vi "温度报警系统（保存到excel）.vi"() -> ()   [LabVIEW 2018]
uses:
  <vilib>/Utility/file.llb/Write Delimited Spreadsheet (string).vi
  <vilib>/Utility/file.llb/Write Delimited Spreadsheet (DBL).vi
panel:
  out "波形图表":dbl(graph)
  out "布尔":bool
  in  "预警值":dbl=50.0
  out "温度计":dbl(slide) scale=0.0..100.0
  in  "停止":bool
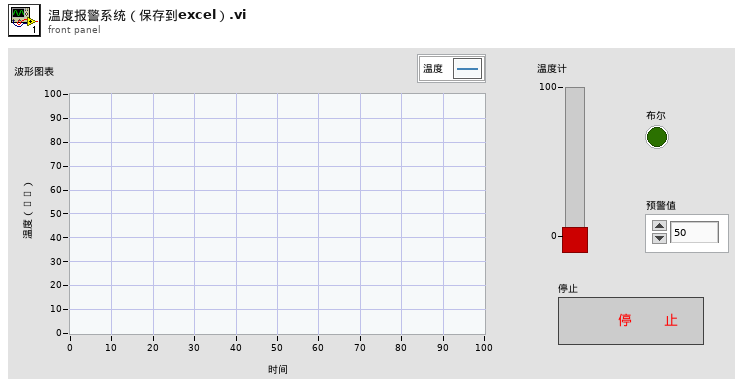
[diagram p1: front panel]
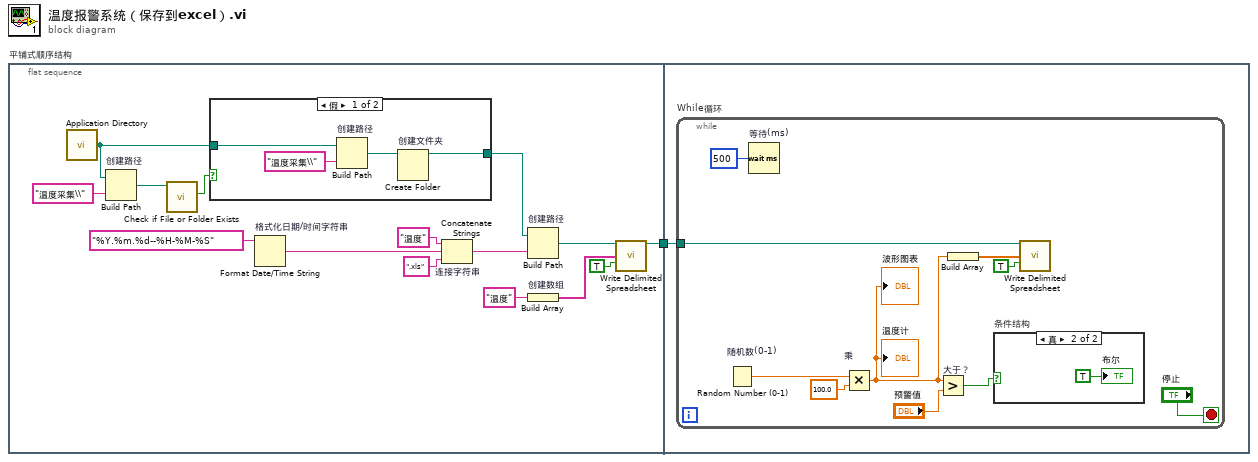
[diagram p0: block diagram]
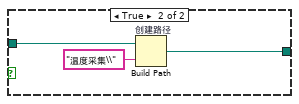
[diagram p2: hidden frame]
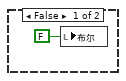
[diagram p3: hidden frame]
diagram:
  n1 = flat-sequence "平铺式顺序结构" {
    tunnel: [w3] -> w1
    tunnel: w1 -> [w24]
    frame #0 {
      n2 = call <vilib>:"Application Directory.vi"() -> ("Application Directory"=w14:path)
      n3 = Build Path "创建路径"(base path=w14, name or relative path="温度采集\\" ("名称或相对路径")) -> (appended path=w12:path)
      n4 = call <vilib>:"Check if File or Folder Exists.vi"("path"=w12) -> ("file or folder exists?"=w13:bool)  [unwired: 8 in, 2 out]
      n5 = case shown="假" w13 {
        tunnel: w14 -> [w20 w23]
        tunnel: [w17 w21] -> w7
        frame False {
          n6 = Build Path "创建路径"(base path=w20, name or relative path="温度采集\\" ("名称或相对路径")) -> (appended path=w18:path)
          n7 = Create Folder "创建文件夹"(path (use dialog)=w18) -> (created path=w17:path)  [unwired: 2 in, 2 out]
        }
        frame True {
          n8 = Build Path "创建路径"(base path=w23, name or relative path="温度采集\\" ("名称或相对路径")) -> (appended path=w21:path)
        }
      }
      n9 = Format Date/Time String "格式化日期/时间字符串"(time format string (%c)="%Y.%m.%d--%H-%M-%S" ("时间格式字符串(%c)")) -> (date/time string=w15:string)  [unwired: 2 in]
      n10 = Concatenate Strings "连接字符串"("温度" ("字符串"), w15, ".xls" ("字符串")) -> (w16:string)
      n11 = Build Path "创建路径"(base path=w7, name or relative path=w16) -> (appended path=w4:path)
      n12 = Build Array "创建数组"("温度" ("字符串")) -> (w5:string[])
      n13 = call-poly <vilib>:"Write Delimited Spreadsheet.vi"("file path (dialog if empty)"=w4, "1D data"=w5, "append to file? (new file:F)"=TRUE) -> ("new file path (Not A Path if cancelled)"=w3:path)  [unwired: 11 in, 1 out]
    }
    frame #1 {
      n14 = while "While循环" {
        tunnel: w24 -> [w28]
        stop <- "停止" stop-if-true
        n15 = Random Number (0-1) "随机数(0-1)"() -> (number: 0 to 1=w32:dbl)
        n16 = Wait (ms) "等待(ms)"(milliseconds to wait=u32 500 ("毫秒计时值")) -> ()  [unwired: 1 out]
        n17 = Multiply "乘"(x=w32, y=100.0) -> (x*y=w27:dbl)
        "温度计" <- w27
        "波形图表" <- w27
        n18 = Greater? "大于？"(x=w27, y="预警值") -> (0:w30:bool)
        n19 = Build Array(w27) -> (w26:dbl[])
        n20 = case "条件结构" shown="真" w30 {
          frame False {
            n21 = local write "布尔"(FALSE ("布尔")) -> ()
          }
          frame True {
            "布尔" <- TRUE ("布尔")
          }
        }
        n22 = call-poly <vilib>:"Write Delimited Spreadsheet.vi"("file path (dialog if empty)"=w28, "1D data"=w26, "append to file? (new file:F)"=TRUE) -> ()  [unwired: 11 in, 2 out]
      }
    }
  }
